vi "BRig_RT_testLoad.vi"() -> ()   [LabVIEW 2014]
panel:
  out "ENL_max":u16
  out "ENL_min":u16
  out "output_dataExp":u16[](array[numeric])
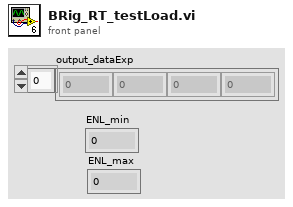
[diagram p1: front panel]
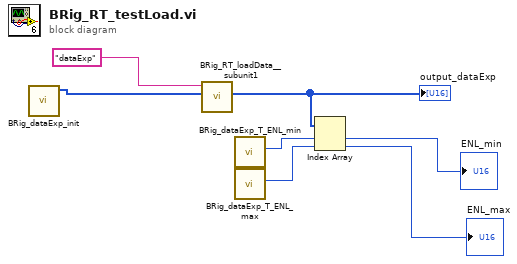
[diagram p0: block diagram]
diagram:
  n1 = call "BRig_dataExp_init.vi"() -> ("output_dataExp"=w6:u16[])  [unwired: 11 in]
  n2 = call "BRig_RT_loadData__subunit1.vi"("input_data"=w6, "input_name"="dataExp" ("string")) -> ("output_data"=w5:u16[])  [unwired: 9 in]
  "output_dataExp" <- w5
  n3 = call "BRig_dataExp_T_ENL_min.vi"() -> ("output_T_ENL_min"=w4:i32)  [unwired: 11 in]
  n4 = call "BRig_dataExp_T_ENL_max.vi"() -> ("output_T_ENL_max"=w3:i32)  [unwired: 11 in]
  n5 = Index Array(array=w5, index #1=w4, index #2=w3) -> (element #1=→"ENL_min":u16, element #2=→"ENL_max":u16)
